vi "Cheby 2D array prep_XY arrays.vi"(5 "Y-array":dbl[](array[numeric]), 6 "X-array":dbl[](array[numeric]), 7 "end":dbl=7.0 format="%.2f", 8 "start":dbl format="%.2f", 9 "order":u32=14) -> (2 "original curve":cluster{dbl[], dbl[]}, 3 "values":dbl[](array[numeric]))   [LabVIEW 2021]
panel:
  out "output cluster":cluster{dbl[], dbl[]}
  out "XY Graph":cluster{dbl[], dbl[]}[](graph)
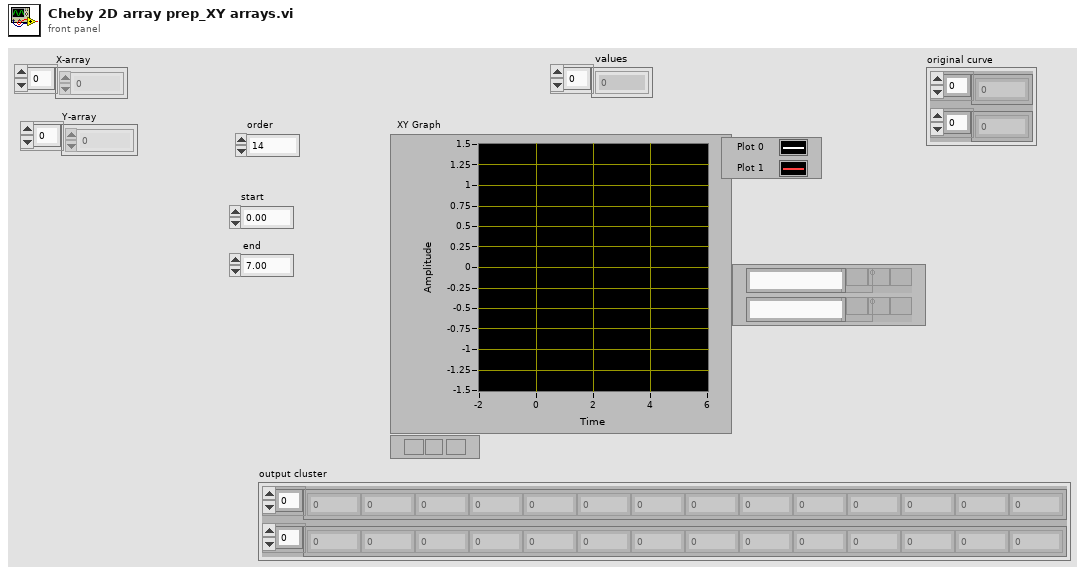
[diagram p1: front panel]
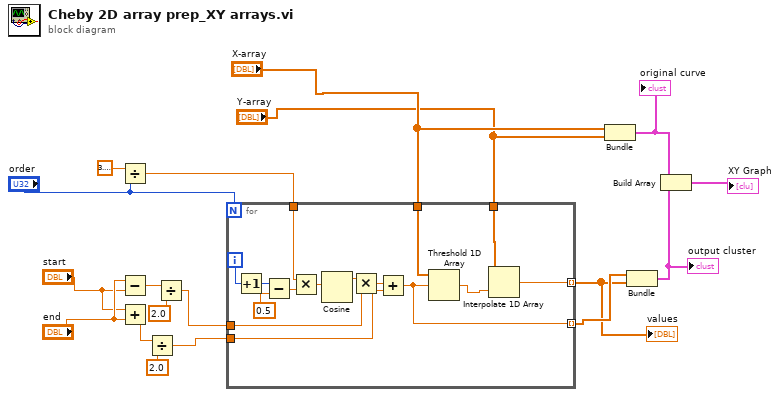
[diagram p0: block diagram]
diagram:
  n1 = Divide(x=3.141592653589793, y="order") -> (x/y=w10:dbl)
  n2 = Subtract(x="end", y="start") -> (x-y=w15:dbl)
  n3 = Add(x="start", y="end") -> (x+y=w17:dbl)
  n4 = Divide(x=w17, y=2.0) -> (x/y=w12:dbl)
  n5 = Divide(x=w15, y=2.0) -> (x/y=w13:dbl)
  n6 = for {
    N: "order" -> [_]
    tunnel: w10 -> [w31]
    tunnel: w13 -> [w27]
    tunnel: w12 -> [w24]
    tunnel: "X-array" -> [w23]
    tunnel: "Y-array" -> [w22]
    tunnel: [w20] -> w3 mode=indexing
    tunnel: [w19] -> w4 mode=indexing
    i -> [w32]
    n7 = Increment(x=w32) -> (x+1=w28:i32)
    n8 = Subtract(x=w28, y=0.5) -> (x-y=w30:dbl)
    n9 = Multiply(x=w31, y=w30) -> (x*y=w29:dbl)
    n10 = Cosine(x=w29) -> (cos(x)=w26:dbl)
    n11 = Multiply(x=w26, y=w27) -> (x*y=w25:dbl)
    n12 = Add(x=w25, y=w24) -> (x+y=w19:dbl)
    n13 = Threshold 1D Array(2:w19, 3:w23) -> (0:w21:dbl)  [unwired: 1 in]
    n14 = Interpolate 1D Array(1:w21, 2:w22) -> (0:w20:dbl)
  }
  "values" <- w3
  n15 = Bundle("X-array"="X-array", "Y-array"="Y-array") -> (w8:cluster{"X-array":dbl[], "Y-array":dbl[]})  [unwired: 1 in]
  "original curve" <- w8
  n16 = Bundle(w4, w3) -> (w9:cluster{dbl[], dbl[]})  [unwired: 1 in]
  "output cluster" <- w9
  n17 = Build Array(w8, w9) -> (→"XY Graph":cluster{"X-array":dbl[], "Y-array":dbl[]}[])
